vi "Read STB w Timeout.vi"(8 "error in (no error)":errorcluster, 10 "STB timeout":u32, 11 "VISA resource name":refnum<visa-resource-name>) -> (0 "error out":errorcluster, 2 "status byte":u16, 3 "VISA resource name out":refnum<visa-resource-name>)   [LabVIEW 2010]
doc: "Copyright (c) 2012 Metrolab Technology SA, Plan-les-Ouates, Geneva, Switzerland\nRead the status byte, with the given timeout value.\nThis VI is only used only as a sub-VI for Write and Read.vi."
panel:
  # "Read STB w Timeout"
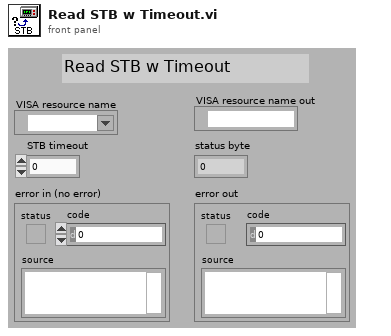
[diagram p1: front panel]
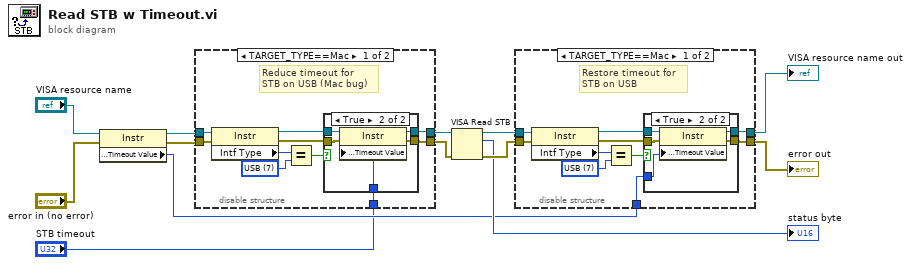
[diagram p0: block diagram]
diagram:
  n1 = property class="Instr"(reference="VISA resource name", error in="error in (no error)") -> (reference out=w3:refnum<visa-resource-name>, error out=w2:errorcluster, "General Settings:Timeout Value"=w4:u32)
  n2 = disable-structure shown="TARGET_TYPE==Mac" {
    disable-tunnel: w2 -> [w17 w31]
    disable-tunnel: w3 -> [w18 w32]
    disable-tunnel: [w15 w31] -> w12
    disable-tunnel: [w16 w32] -> w13
    disable-tunnel: "STB timeout" -> [w14 _]
    frame condition #0 (active) {
      w19 = u16 7 items=["GPIB"=1, "VXI"=2, "GPIB-VXI"=3, "Serial"=4, "PXI"=5, "TCPIP"=6, "USB"=7, "FireWire"=9] ("Interface Information:Interface Type")
      # "Reduce timeout for\nSTB on USB (Mac bug)"
      n3 = property class="Instr"(reference=w18, error in=w17) -> (reference out=w22:refnum<visa-resource-name>, error out=w23:errorcluster, "Intf Type"=w20:u16)
      n4 = Equal?(x=w20, y=w19) -> (x = y?=w21:bool)
      n5 = case shown="True" w21 {
        tunnel: w22 -> [w25 w30]
        tunnel: w23 -> [w24 w29]
        tunnel: [w25 w28] -> w16
        tunnel: [w24 w27] -> w15
        tunnel: w14 -> [_ w26]
        frame False {
        }
        frame True {
          n6 = property class="Instr"(reference=w30, error in=w29, "General Settings:Timeout Value"=w26) -> (reference out=w28:refnum<visa-resource-name>, error out=w27:errorcluster)
        }
      }
    }
    frame condition #1 {
    }
  }
  n7 = VISA Read STB(8:w12, 11:w13) -> (0:w10:errorcluster, 2:→"status byte":u16, 3:w11:refnum<visa-resource-name>)
  n8 = disable-structure shown="TARGET_TYPE==Mac" {
    disable-tunnel: w10 -> [w36 w50]
    disable-tunnel: w11 -> [w37 w51]
    disable-tunnel: [w34 w50] -> w7
    disable-tunnel: [w35 w51] -> w8
    disable-tunnel: w4 -> [w33 _]
    frame condition #0 (active) {
      w38 = u16 7 items=["GPIB"=1, "VXI"=2, "GPIB-VXI"=3, "Serial"=4, "PXI"=5, "TCPIP"=6, "USB"=7, "FireWire"=9] ("Interface Information:Interface Type")
      # "Restore timeout for\nSTB on USB"
      n9 = property class="Instr"(reference=w37, error in=w36) -> (reference out=w41:refnum<visa-resource-name>, error out=w42:errorcluster, "Intf Type"=w39:u16)
      n10 = Equal?(x=w39, y=w38) -> (x = y?=w40:bool)
      n11 = case shown="True" w40 {
        tunnel: w41 -> [w44 w49]
        tunnel: w42 -> [w43 w48]
        tunnel: [w44 w47] -> w35
        tunnel: [w43 w46] -> w34
        tunnel: w33 -> [_ w45]
        frame False {
        }
        frame True {
          n12 = property class="Instr"(reference=w49, error in=w48, "General Settings:Timeout Value"=w45) -> (reference out=w47:refnum<visa-resource-name>, error out=w46:errorcluster)
        }
      }
    }
    frame condition #1 {
    }
  }
  "error out" <- w7
  "VISA resource name out" <- w8
